vi "CTI_AOTFQSM.vi"(10 "error in (no error)":errorcluster) -> ()   [LabVIEW 2011]
uses:
  Utilities/controls/ctlSeqFNs_AVTGuppy.ctl
  Utilities/controls/ctlSeqFNs_CTIOTF.ctl
  Utilities/controls/ctlSeqFNs_PCDeviceInit.ctl
  Utilities/controls/ctlSeqFNs_Main.ctl
  <vilib>/userDefined/High Color/IMAQdx.ctl
panel:
  in  "config remote device":T2
  in  "CTIOTF Vals":cluster{bool[], i32[], i16[]}={[FALSE, FALSE, FALSE, FALSE, FALSE, FALSE, FALSE, FALSE], [0, 0, 0, 0, 0, 0, 0, 0], [0, 0, 0, 0, 0, 0, 0, 0]}
  in  "Config Out ctiotf":string[](array[string])
  in  "remote device online status":T3
  in  "interface management remote device":T4
  in  "set remote device online":T3
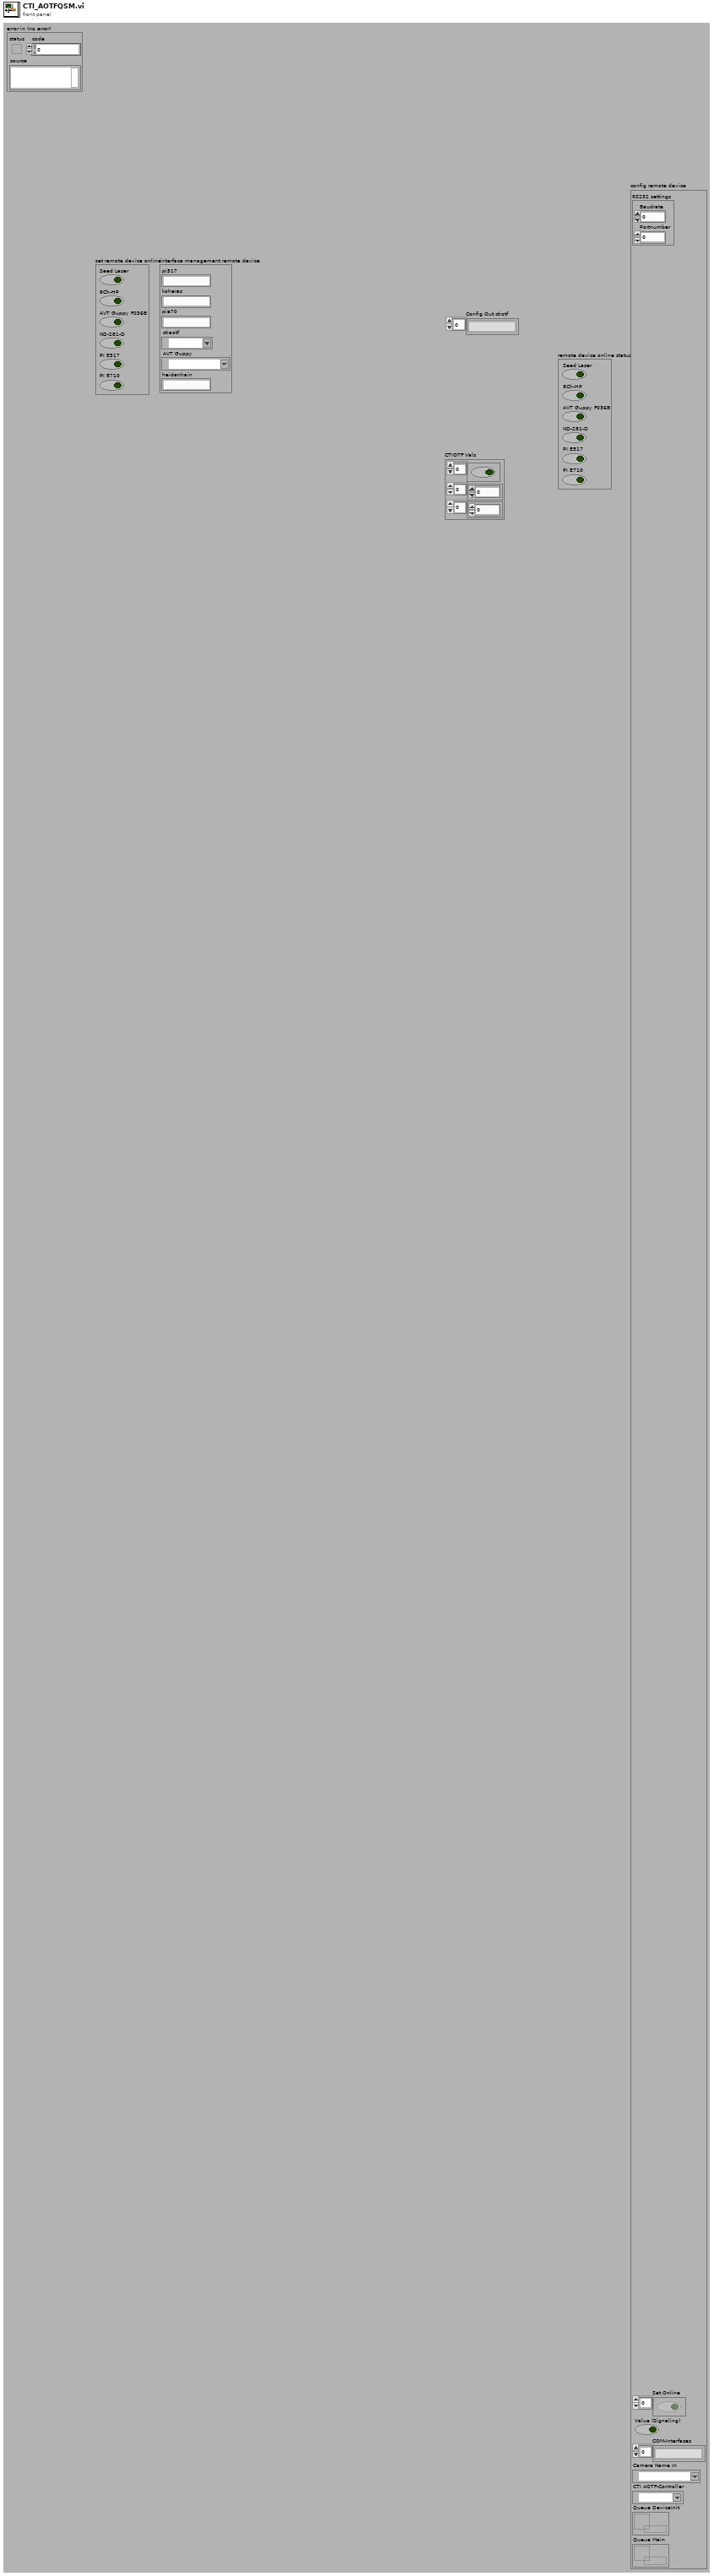
[diagram p1: front panel]
types:
  T1 = typedef "IMAQdx.ctl" = refnum<k21>
  T2 = cluster{"RS232 settings":cluster{"Baudrate":u16, "Portnumber":i32}, "Set Online":bool[], "Value (Signaling)":bool, "COM-Interfaces":string[], "Camera Name In":T1, "CTI AOTF-Controller":refnum<visa-resource-name>, "Queue DeviceInit":refnum<queue>, "Queue Main":refnum<queue>}
  T3 = cluster{"Seed Laser":bool, "8Ch-HP":bool, "AVT Guppy F036B":bool, "ND-281-D":bool, "PI E517":bool, "PI E710":bool}
  T4 = cluster{"pi517":string, "koheras":string, "pie70":string, "ctiaotf":refnum<visa-resource-name>, "AVT Guppy":T1, "heidenhain":string}
  T5 = typedef "ctlSeqFNs_CTIOTF.ctl" = enum16{"ERROR", "INIT", "Initialization", "Configuration", "Measurement", "Shutdown", "IDLE", "EXIT"}
  T6 = cluster{"Queue DeviceInit":refnum<queue>, "CTIOTF Vals":cluster{bool[], i32[], i16[]}, "Config Out ctiotf":string[], "set remote device online":cluster{"Seed Laser":bool, "8Ch-HP":bool, "AVT Guppy F036B":bool, "ND-281-D":bool, "PI E517":bool, "PI E710":bool}, "config remote device":cluster{"RS232 settings":cluster{"Baudrate":u16, "Portnumber":i32}, "Set Online":bool[], "Value (Signaling)":bool, "COM-Interfaces":string[], "Camera Name In":T1, "CTI AOTF-Controller":refnum<visa-resource-name>, "Queue DeviceInit":refnum<queue>, "Queue Main":refnum<queue>}, "remote device online status":cluster{"Seed Laser":bool, "8Ch-HP":bool, "AVT Guppy F036B":bool, "ND-281-D":bool, "PI E517":bool, "PI E710":bool}, "interface management remote device":cluster{"pi517":string, "koheras":string, "pie70":string, "ctiaotf":refnum<visa-resource-name>, "AVT Guppy":T1, "heidenhain":string}}
  T7 = typedef "ctlSeqFNs_AVTGuppy.ctl" = enum16{"ERROR", "INIT", "Initialization", "Configuration", "Measurement", "Shutdown", "IDLE", "EXIT"}
  T8 = typedef "ctlSeqFNs_PCDeviceInit.ctl" = enum16{"ERROR", "INIT", "ErrorDevice", "StartDevice", "DeviceStatus", "StopDevice", "EXIT", "IDLE"}
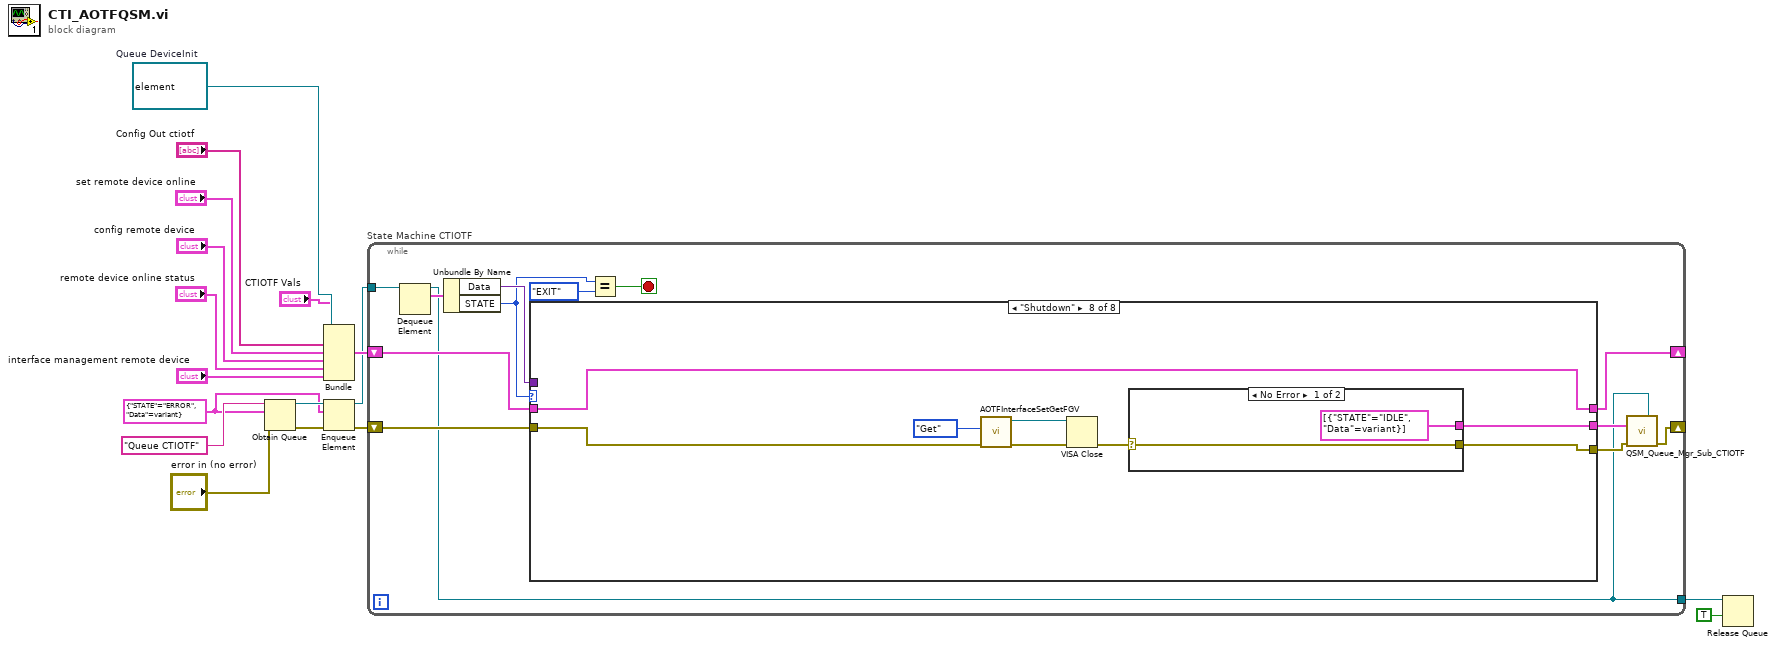
[diagram p0: block diagram]
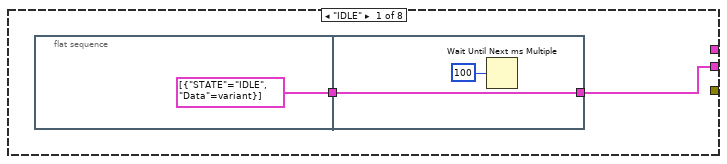
[diagram p2: hidden frame]
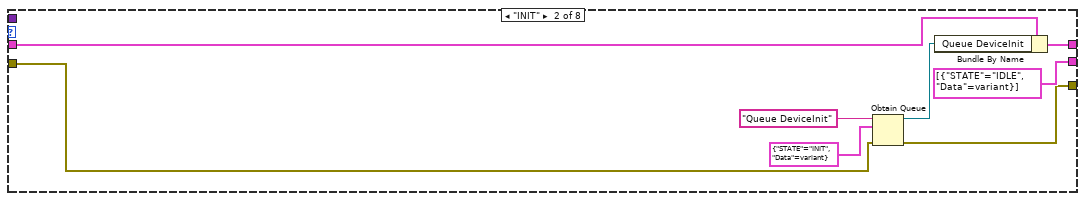
[diagram p3: hidden frame]
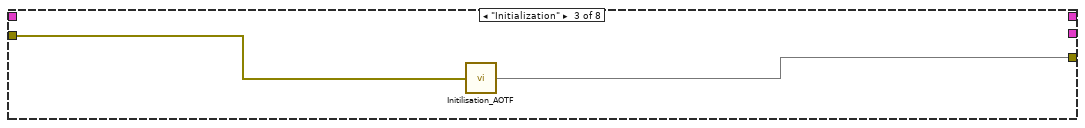
[diagram p4: hidden frame]
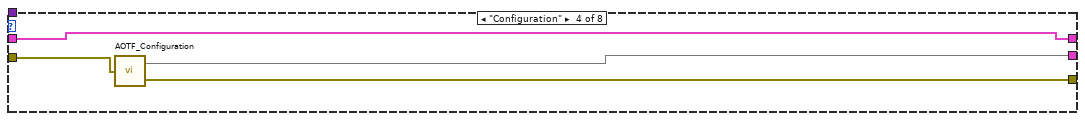
[diagram p5: hidden frame]
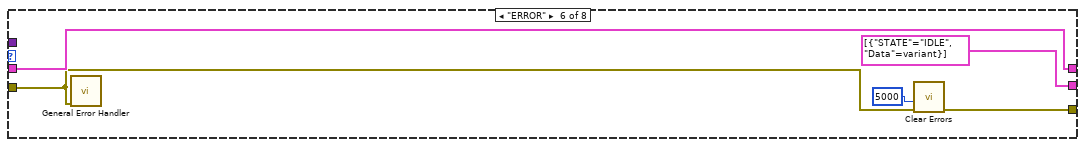
[diagram p7: hidden frame]
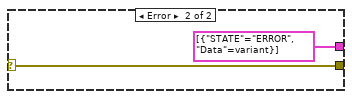
[diagram p9: hidden frame]
diagram:
  w4 = refnum<queue> refnum  # Queue DeviceInit
  w9 = cluster{"STATE":T5, "Data":variant} {"STATE"=enum."ERROR", "Data"=variant} ("element")
  n1 = Obtain Queue(name (unnamed)="Queue CTIOTF", element data type=w9, error in (no error)="error in (no error)") -> (queue out=w14:refnum<queue>, error out=w16:errorcluster)  [unwired: 2 in, 1 out]
  n2 = Bundle("Queue DeviceInit"=w4, "CTIOTF Vals"="CTIOTF Vals", "Config Out ctiotf"="Config Out ctiotf", "set remote device online"="set remote device online", "config remote device"="config remote device", "remote device online status"="remote device online status", "interface management remote device"="interface management remote device") -> (w13:T6)  [unwired: 1 in]
  n3 = Enqueue Element(queue=w14, element=w9, error in (no error)=w16) -> (queue out=w10:refnum<queue>, error out=w15:errorcluster)  [unwired: 1 in, 1 out]
  n4 = while "State Machine CTIOTF" {
    shift-right: [w19] -> _
    shift-left: w15 -> [w30]
    tunnel: w10 -> [w28]
    tunnel: [w18] -> w12
    shift-right: [w23] -> _
    shift-left: w13 -> [w24]
    stop <- w29 stop-if-true
    n5 = Dequeue Element(queue=w28) -> (queue out=w18:refnum<queue>, element=w27:cluster{"STATE":T5, "Data":variant})  [unwired: 2 in, 2 out]
    n6 = Unbundle By Name(w27) -> ("Data"=w26:variant, "STATE"=w25:T5)
    n7 = case shown="\"Shutdown\"" w25 {
      tunnel: w30 -> [_ w37 w45 w46 w50 w54 w57 w62]
      tunnel: w26 -> [_ _ _ _ _ _ _ _]
      tunnel: w24 -> [_ w41 _ w49 w51 w56 w58 w66]
      tunnel: [_ w40 _ w49 w51 w56 w58 w66] -> w23
      tunnel: [w31 cluster{"STATE":T5, "Data":variant}[] [{"STATE"=enum."IDLE", "Data"=variant}] ("QFNs") _ w48 _ cluster{"STATE":T5, "Data":variant}[] [{"STATE"=enum."IDLE", "Data"=variant}] ("QFNs") _ w63] -> w21
      tunnel: [_ w36 w44 w47 w50 w53 w57 w64] -> w20
      frame "IDLE" {
        n8 = flat-sequence {
          tunnel: [cluster{"STATE":T5, "Data":variant}[] [{"STATE"=enum."IDLE", "Data"=variant}] ("QFNs")] -> w32
          tunnel: w32 -> [w34]
          tunnel: [w34] -> w31
          frame #0 {
          }
          frame #1 {
            n9 = Wait Until Next ms Multiple(millisecond multiple=u32 100) -> ()  [unwired: 1 out]
          }
        }
      }
      frame "INIT" {
        n10 = Obtain Queue(name (unnamed)="Queue DeviceInit" ("Queue Name"), element data type=cluster{"STATE":T8, "Data":variant} {"STATE"=enum."INIT", "Data"=variant} ("element"), error in (no error)=w37) -> (queue out=w39:refnum<queue>, error out=w36:errorcluster)  [unwired: 2 in, 1 out]
        n11 = Bundle By Name(cluster=w41, "Queue DeviceInit"=w39) -> (w40:T6)
      }
      frame "Initialization" {
        n12 = call "Initilisation_AOTF.vi"(1:w45) -> (0:w44)
      }
      frame "Configuration" {
        n13 = call "AOTF_Configuration.vi"("error out"=w46) -> ("error out 2"=w47:errorcluster, 2:w48)
      }
      frame "Measurement" {
      }
      frame "ERROR" {
        n14 = call <vilib>:"General Error Handler.vi"("error in (no error)"=w54) -> ()  [unwired: 10 in, 5 out]
        n15 = call <vilib>:"Clear Errors.vi"("error in (no error)"=w54, 5:u32 5000 ("wait(ms)")) -> ("error out"=w53:errorcluster)  [unwired: 5 in]
      }
      frame "EXIT" {
      }
      frame "Shutdown" {
        n16 = call "AOTFInterfaceSetGetFGV.vi"("error in"=w62, "FGV_Control"=enum16{"Set", "Get"}."Get") -> ("error out"=w61:errorcluster, "ctiaotf interface get"=w60:refnum<visa-resource-name>)  [unwired: 8 in]
        n17 = VISA Close(VISA resource name=w60, error in (no error)=w61) -> (error out=w65:errorcluster)
        n18 = case shown="No Error" w65 {
          selector: w65 -> [w68 w70]
          tunnel: [w68 w70] -> w64
          tunnel: [cluster{"STATE":T5, "Data":variant}[] [{"STATE"=enum."IDLE", "Data"=variant}] ("QFNs") cluster{"STATE":T5, "Data":variant}[] [{"STATE"=enum."ERROR", "Data"=variant}] ("QFNs")] -> w63
          frame No Error {
          }
          frame Error {
          }
        }
      }
    }
    n19 = Equal?(x=w25, y=ctlSeqFNs_AVTGuppy."EXIT" ("STATE")) -> (x = y?=w29:bool)
    n20 = call "QSM_Queue_Mgr_Sub_CTIOTF.vi"("QRef"=w18, "QSTATES"=w21, "Error IN"=w20) -> ("Error OUT"=w19:errorcluster)  [unwired: 12 in]
  }
  n21 = Release Queue(queue=w12, force destroy? (F)=TRUE) -> ()  [unwired: 1 in, 3 out]
